vi "ProcessInput.vi"(8 "Error In (no error)":errorcluster, 10 "TeleopData":T1) -> (0 "Error Out":errorcluster)   [LabVIEW 2012]
doc: "Takes data from teleop and determines what instructions, if any, need to be enqueued."
uses:
  TeleopData.ctl
  Robot Global Data.vi
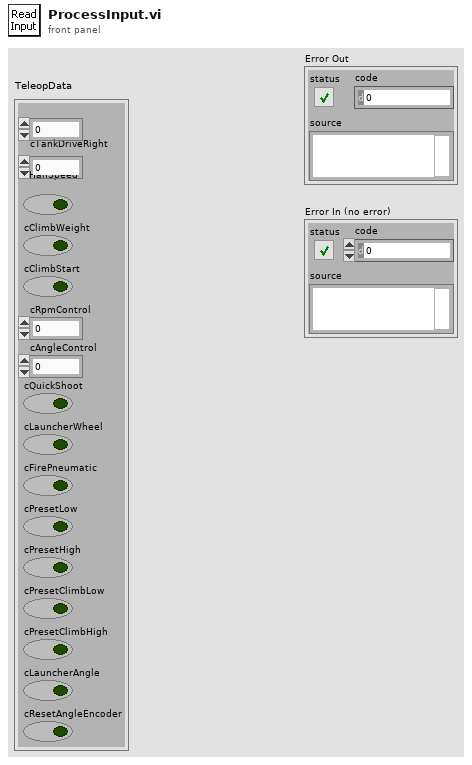
[diagram p1: front panel]
types:
  T1 = typedef "TeleopData.ctl" = cluster{"cTankDriveLeft":dbl, "cTankDriveRight":dbl, "cHalfSpeed":bool, "cClimbWeight":bool, "cClimbStart":bool, "cRpmControl":dbl, "cAngleControl":dbl, "cQuickShoot":bool, "cLauncherWheel":bool, "cFirePneumatic":bool, "cPresetLow":bool, "cPresetHigh":bool, "cPresetClimbLow":bool, "cPresetClimbHigh":bool, "cLauncherAngle":bool, "cResetAngleEncoder":bool}
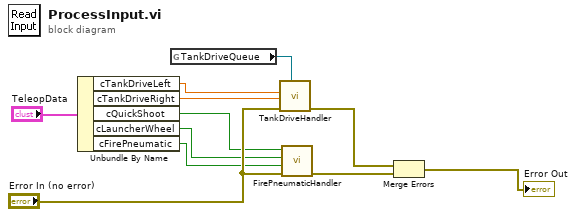
[diagram p0: block diagram]
diagram:
  n1 = Unbundle By Name("TeleopData") -> ("cTankDriveLeft"=w10:dbl, "cTankDriveRight"=w9:dbl, "cQuickShoot"=w1:bool, "cLauncherWheel"=w2:bool, "cFirePneumatic"=w3:bool)
  n2 = global read "Robot Global Data.vi" "TankDriveQueue"() -> (w4:refnum<queue>)
  n3 = call "TankDriveHandler.vi"("TankDrive Queue"=w4, "Error In (no error)"="Error In (no error)", "Right Motor Value"=w9, "Left Motor Value"=w10) -> ("Error Out"=w7:errorcluster)  [unwired: 7 in]
  n4 = call "FirePneumaticHandler.vi"("error in (no error)"="Error In (no error)", "cFirePneumatic"=w3, "cLauncherWheel"=w2, "cQuickShoot"=w1) -> ("error out"=w6:errorcluster)  [unwired: 7 in]
  n5 = Merge Errors(w7, w6) -> (→"Error Out":errorcluster)
